vi "FTW-TestExecutive-Core_Step_Complete.vi"(0 "FTW-TestExecutive-Core In":refnum<class "FTW-TestExecutive-Core.lvclass">, 7 "Results":T1 {"Start Time" format="%<%Y-%m-%d %H:%M:%S%03u>T"; "Elapsed Time" format="%<%H:%M:%S%3u>t"}, 11 "error in":errorcluster) -> (4 "FTW-TestExecutive-Core Out":refnum<class "FTW-TestExecutive-Core.lvclass">, 15 "error out":errorcluster)   [LabVIEW 2015, in "FTW-TestExecutive-Core.lvclass"]
uses:
  FTW-TestExecutive-Core.lvclass
  FTW-TestExecutive-Results.ctl
  FTW-TestExecutive-Step-State.ctl
  FTW-TestExecutive-Core.lvclass/FTW-TestExecutive-Core.ctl
  FTW-TestExecutive-Core_State.ctl
  Connector/FTW-ActorConnector.lvclass
  Instance/FTW-ActorInstance.lvclass
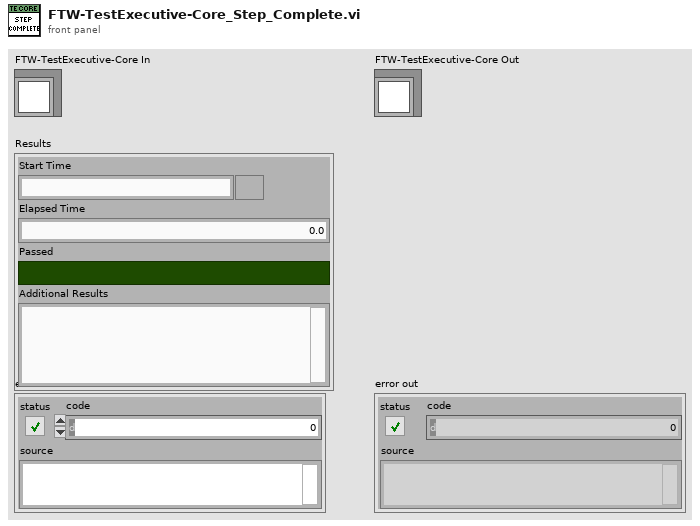
[diagram p1: front panel]
types:
  T1 = typedef "FTW-TestExecutive-Results.ctl" = cluster{"Start Time":timestamp, "Elapsed Time":dbl, "Passed":bool, "Additional Results":string}
  T2 = typedef "FTW-TestExecutive-Step-State.ctl" = enum8{"None", "Failed", "Passed", "Timed out", "Aborted"}
  T3 = typedef "FTW-TestExecutive-Core.lvclass/FTW-TestExecutive-Core_State.ctl" = enum8{"Unloaded", "Loaded", "Executing", "Paused"}
  T4 = typedef "FTW-TestExecutive-Step.ctl" = cluster{"Name":string, "Type":string, "Config":string, "Elapsed Time":dbl, "Passed":bool, "State":T2, "Results":T1}
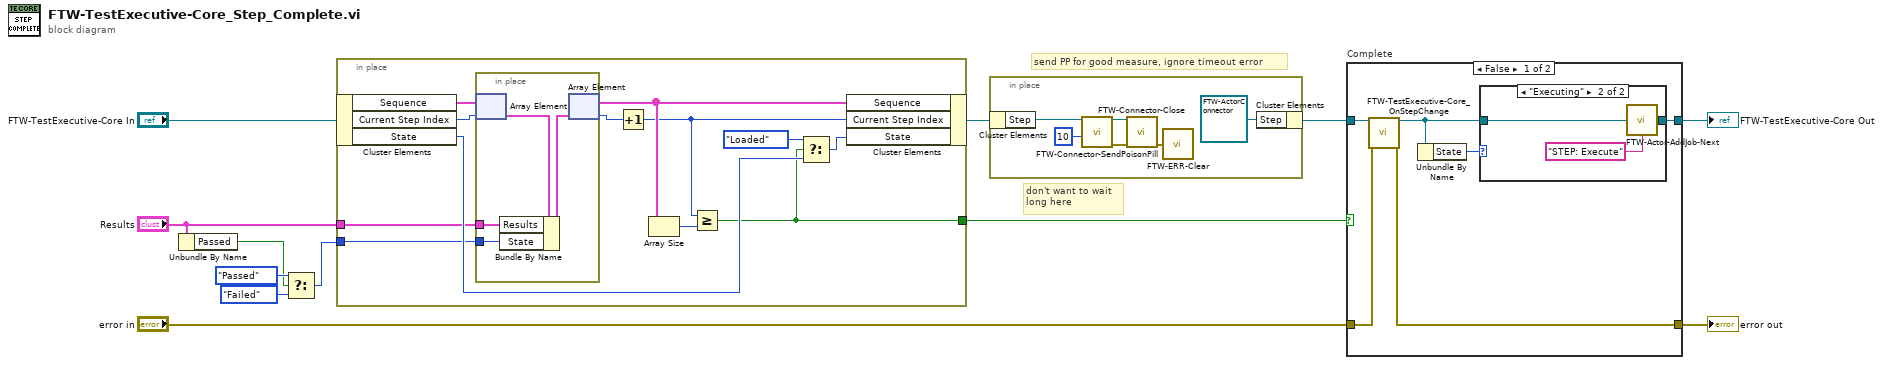
[diagram p0: block diagram]
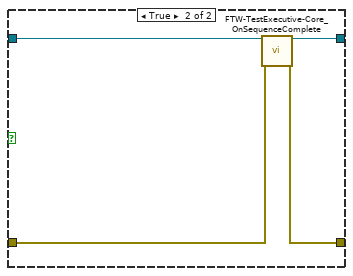
[diagram p3: hidden frame]
diagram:
  # "send PP for good measure, ignore timeout error"
  # "don't want to wait\nlong here"
  n1 = Unbundle By Name("Results") -> ("Passed"=w7:bool)
  n2 = Select(t=FTW-TestExecutive-Step-State."Passed" ("State"), s=w7, f=FTW-TestExecutive-Step-State."Failed") -> (s? t:f=w10:T2)
  n3 = in-place {
    in-place-border: "Results" -> [w21]
    in-place-border: w10 -> [w20]
    in-place-border: [w13] -> w4
    n4 = in-place-cluster #1("FTW-TestExecutive-Core In") -> ("Sequence"=w22:T4[], "Current Step Index"=w19:i32, "State"=w24:T3)
    n5 = in-place {
      in-place-border: w21 -> [w26]
      in-place-border: w20 -> [w25]
      n6 = in-place-array #2(w22, w19) -> (w28:T4)
      n7 = Bundle By Name(cluster=w28, "Results"=w26, "State"=w25) -> (w27:T4)
      n8 = in-place-array #2(w27) -> (w23:T4[], w18:i32)
    }
    n9 = Increment(x=w18) -> (x+1=w17:i32)
    n10 = Array Size(array=w23) -> (size(s)=w16:i32)
    n11 = Greater Or Equal?(x=w17, y=w16) -> (x >= y?=w13:bool)
    n12 = Select(t=FTW-TestExecutive-Core_State."Loaded" ("State"), s=w13, f=w24) -> (s? t:f=w14:T3)
    n13 = in-place-cluster #1("Sequence"=w23, "Current Step Index"=w17, "State"=w14) -> (w2:refnum<class "FTW-TestExecutive-Core.lvclass">)
  }
  n14 = in-place {
    n15 = in-place-cluster #3(w2) -> ("Step"=w31:refnum<class "FTW-ActorConnector.lvclass">)
    n16 = call-dynamic "FTW-Connector-SendPoisonPill.vi"("FTW Actor Connector"=w31, "Timeout"=10) -> ("FTW Actor Connector out"=w34:refnum<class "FTW-ActorConnector.lvclass">, "error out"=w33:errorcluster)  [unwired: 8 in, 4 out]
    n17 = call-dynamic "FTW-Connector-Close.vi"("FTW Actor Connector"=w34, "error in"=w33) -> ("error out"=w29:errorcluster)  [unwired: 13 in]
    n18 = call "FTW-ERR-Clear.vi"("error to snuff"=w29) -> ()  [unwired: 1 out]
    n19 = in-place-cluster #3("Step"=refnum<class "FTW-ActorConnector.lvclass"> refnum) -> (w1:refnum<class "FTW-TestExecutive-Core.lvclass">)
  }
  n20 = case "Complete" shown="False" w4 {
    tunnel: w1 -> [w40 w48]
    tunnel: [w39 w47] -> w6
    tunnel: "error in" -> [w38 w46]
    tunnel: [w37 w45] -> w5
    frame False {
      n21 = call "FTW-TestExecutive-Core_OnStepChange.vi"("FTW-TestExecutive-Core In"=w40, "error in"=w38) -> ("FTW-TestExecutive-Core Out"=w36:refnum<class "FTW-TestExecutive-Core.lvclass">, "error out"=w37:errorcluster)  [unwired: 12 in]
      n22 = Unbundle By Name(w36) -> ("State"=w35:T3)
      n23 = case shown="\"Executing\"" w35 {
        tunnel: w36 -> [w41 w44]
        tunnel: [w41 w43] -> w39
        frame "Unloaded", "Loaded", "Paused" {
        }
        frame "Executing" {
          n24 = call "FTW-Actor-AddJob-Next.vi"("Add Next in Job Queue"="STEP: Execute", "FTW Actor Instance"=w44) -> ("FTW Actor Instance out"=w43:refnum<class "FTW-TestExecutive-Core.lvclass">)  [unwired: 2 in]
        }
      }
    }
    frame True {
      n25 = call "FTW-TestExecutive-Core_OnSequenceComplete.vi"("FTW-TestExecutive-Core In"=w48, "error in"=w46) -> ("FTW-TestExecutive-Core Out"=w47:refnum<class "FTW-TestExecutive-Core.lvclass">, "error out"=w45:errorcluster)  [unwired: 12 in]
    }
  }
  "FTW-TestExecutive-Core Out" <- w6
  "error out" <- w5
